vi "Destroy.vi"(8 "error in (no error)":errorcluster, 11 "Element in":refnum<class "Element.lvclass">) -> (0 "error out":errorcluster)   [LabVIEW 2021, in "Element.lvclass"]
uses:
  Element.lvclass
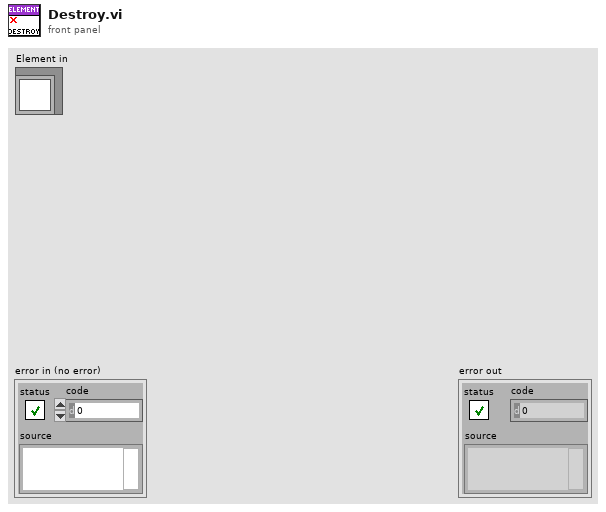
[diagram p1: front panel]
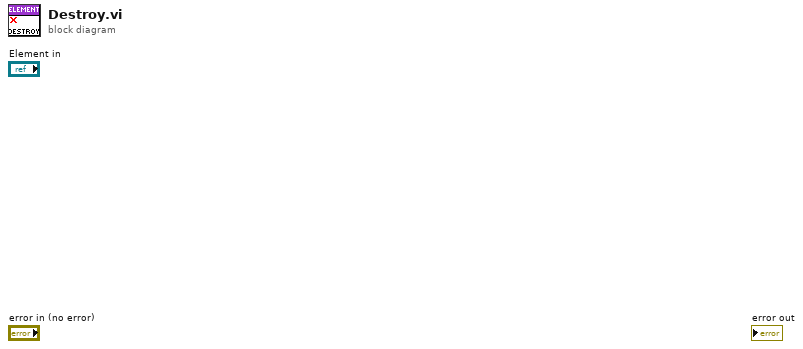
[diagram p0: block diagram]
diagram:
